vi "JKI-easyXML Test Marshall-Unmarshall.vi"() -> ()   [LabVIEW 2019]
uses:
  jki-json/unittests/Test Cluster.ctl
  source/Serializer.easyXML.lvclass
  C:/Program Files (x86)/National Instruments/LabVIEW 2019/vi.lib/LabVIEW Open Source Project/OpenSerializer/Serializer/Serializer.lvclass
  <vilib>/LabVIEW Open Source Project/OpenSerializer/Serializer/Serializer.lvclass
panel:
  out "error out":errorcluster
  out "Pass?":bool
  out "Data Cluster out":T1={"Top-Level"={"Boolean"=FALSE, "String"="", "Path"=path "", "Numeric"=0.0, "Enum"=enum."Item0", "Array"=[], "Sub-Cluster"={"Numeric"=0.0, "Boolean"=FALSE, "Empty String"=""}, "Multi-Line String"=""}} {"Top-Level"."Numeric" format="%#_10g"}
  out "JSON String":string
  in  "Data Cluster in":T1={"Top-Level"={"Boolean"=FALSE, "String"="Another test string", "Path"=path "C:/Windows", "Numeric"=4.0, "Enum"=enum."Item0", "Array"=[0.0, 1.0, 2.0, 3.0, 4.0, 5.0, 6.0], "Sub-Cluster"={"Numeric"=0.0, "Boolean"=TRUE, "Empty String"="Test String Here"}, "Multi-Line String"="Test String Here\nLine2\nLine3"}} {"Top-Level"."Numeric" format="%#_10g"}
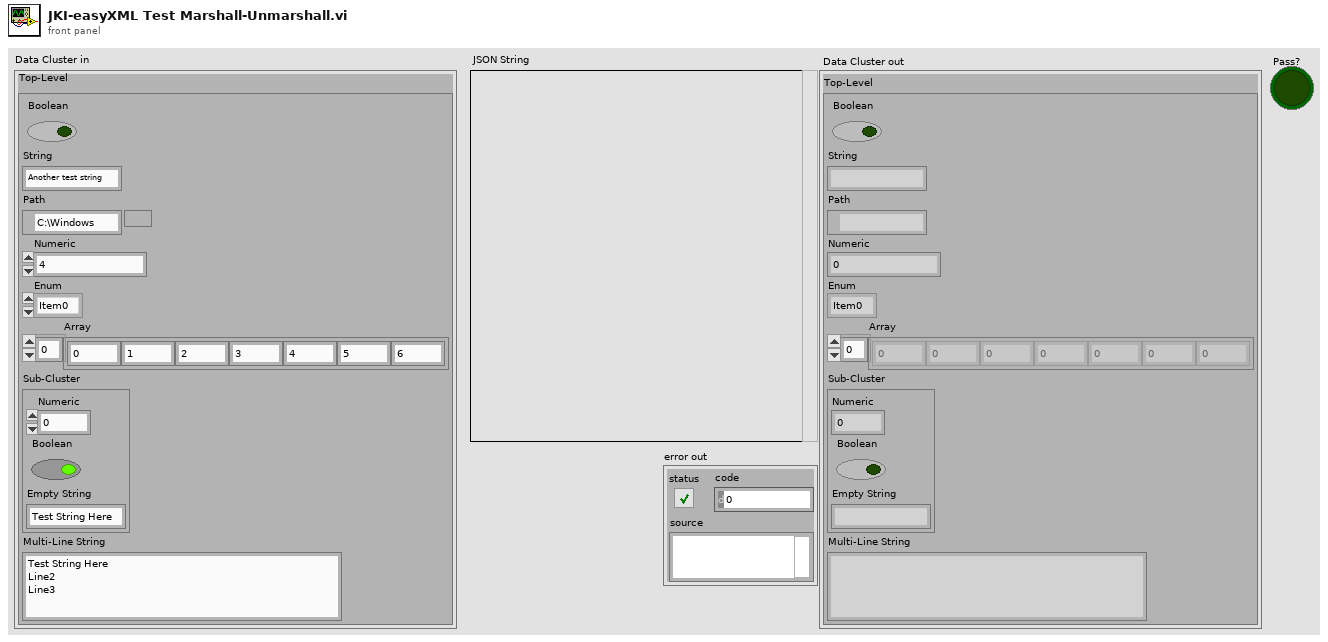
[diagram p1: front panel]
types:
  T1 = typedef "Test Cluster.ctl" = cluster{"Top-Level":cluster{"Boolean":bool, "String":string, "Path":path, "Numeric":dbl, "Enum":enum16{"Item0", "Item1"}, "Array":dbl[], "Sub-Cluster":cluster{"Numeric":dbl, "Boolean":bool, "Empty String":string}, "Multi-Line String":string}}
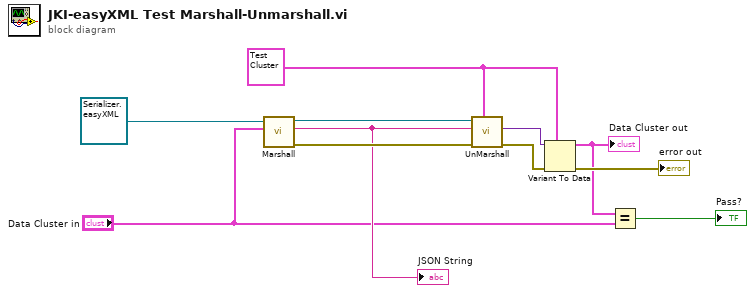
[diagram p0: block diagram]
diagram:
  w7 = T1 {"Top-Level"={"Boolean"=FALSE, "String"="", "Path"=path "", "Numeric"=0.0, "Enum"=enum."Item0", "Array"=[], "Sub-Cluster"={"Numeric"=0.0, "Boolean"=FALSE, "Empty String"=""}, "Multi-Line String"="Test String Here\nLine2\nLine3"}} ("Cluster")
  n1 = call <vilib>:"Marshall.vi"("Variant"="Data Cluster in", "Serializer in"=refnum<class "Serializer.easyXML.lvclass"> refnum ("OpenSerializer.easyXML.lvlib:Serializer.easyXML.lvclass")) -> ("error out"=w11:errorcluster, "String"=w6:string, "Serializer out"=w10:refnum<class "Serializer.easyXML.lvclass">)  [unwired: 7 in]
  "JSON String" <- w6
  n2 = call <vilib>:"UnMarshall.vi"("Type"=w7, "error in (no error)"=w11, "String"=w6, "Serializer in"=w10) -> ("error out"=w9:errorcluster, "Variant"=w8:variant)  [unwired: 5 in, 1 out]
  n3 = Variant To Data(error in=w9, type=w7, Variant=w8) -> (data=w4:T1, error out=→"error out":errorcluster)
  "Data Cluster out" <- w4
  n4 = Equal?(x=w4, y="Data Cluster in") -> (x = y?=→"Pass?":bool)
